vi "Color to Display.vi"(11 "Color state":T2) -> (3 "Traffic Lights":T1)   [LabVIEW 2018]
uses:
  Color states.ctl
  Lights Display.ctl
panel:
  in  "Time scale":dbl
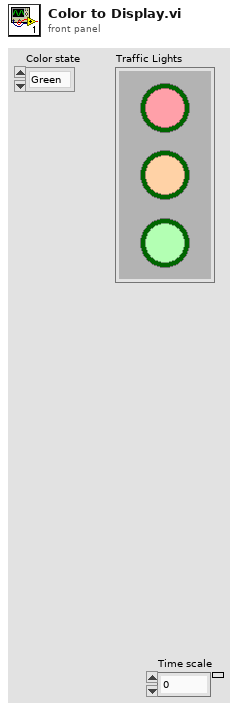
[diagram p1: front panel]
types:
  T1 = typedef "Lights Display.ctl" = cluster{"Red":bool, "Amber":bool, "Green":bool}
  T2 = typedef "Color states.ctl" = enum16{"Green", "Red-Yellow", "Yellow", "Red", "Null"}
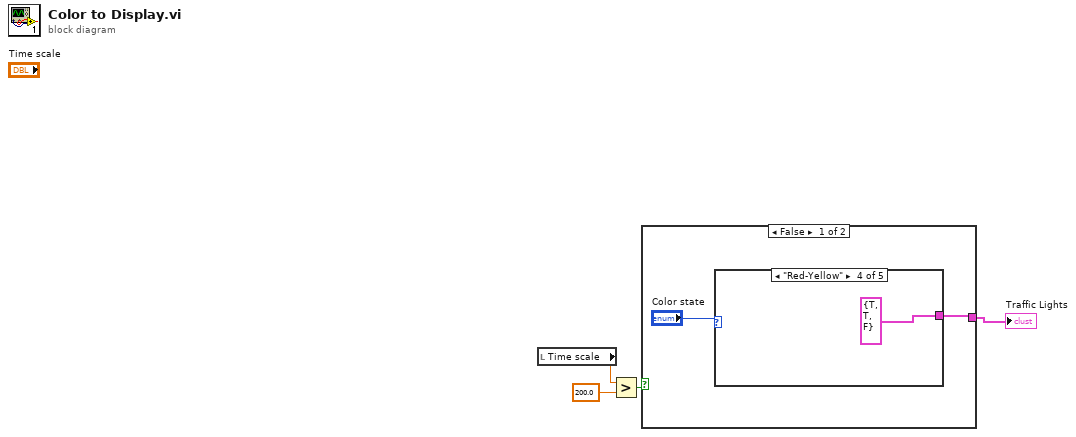
[diagram p0: block diagram]
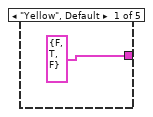
[diagram p2: hidden frame]
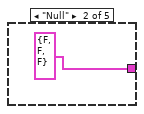
[diagram p3: hidden frame]
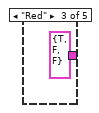
[diagram p4: hidden frame]
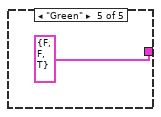
[diagram p5: hidden frame]
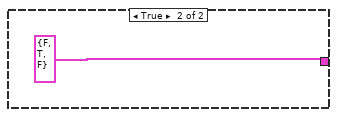
[diagram p6: hidden frame]
diagram:
  n1 = local read "Time scale"() -> (w2:dbl)
  n2 = Greater?(x=w2, y=200.0) -> (0:w4:bool)
  n3 = case shown="False" w4 {
    tunnel: [w5 T1 {"Red"=FALSE, "Amber"=TRUE, "Green"=FALSE} ("Traffic Lights")] -> w1
    frame False {
      n4 = case shown="\"Red-Yellow\"" "Color state" {
        tunnel: [T1 {"Red"=FALSE, "Amber"=TRUE, "Green"=FALSE} ("Traffic Lights") T1 {"Red"=FALSE, "Amber"=FALSE, "Green"=FALSE} ("Traffic Lights") T1 {"Red"=TRUE, "Amber"=FALSE, "Green"=FALSE} ("Traffic Lights") T1 {"Red"=TRUE, "Amber"=TRUE, "Green"=FALSE} ("Traffic Lights") T1 {"Red"=FALSE, "Amber"=FALSE, "Green"=TRUE} ("Traffic Lights")] -> w5
        frame "Yellow", Default {
        }
        frame "Null" {
        }
        frame "Red" {
        }
        frame "Red-Yellow" {
        }
        frame "Green" {
        }
      }
    }
    frame True {
    }
  }
  "Traffic Lights" <- w1
